vi "Read Data Type Handler Type.vi"(11 "ITest Executive Builder Dialog in":refnum<class "ITest Executive Builder Dialog.lvclass">) -> (3 "ITest Executive Builder Dialog out":refnum<class "ITest Executive Builder Dialog.lvclass">, 4 "Data Type Handler":refnum<class "Test Executive Builder Data Type Handler.lvclass">)   [LabVIEW 2017, in "ITest Executive Builder Dialog.lvclass"]
uses:
  ITest Executive Builder Dialog.lvclass
  Data Type Handler/Test Executive Builder Data Type Handler.lvclass
  ITest Executive Builder Dialog.lvclass/ITest Executive Builder Dialog.ctl
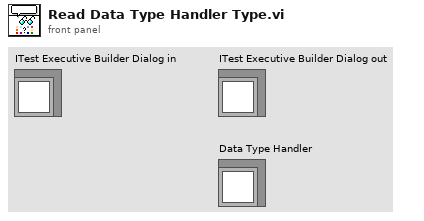
[diagram p1: front panel]
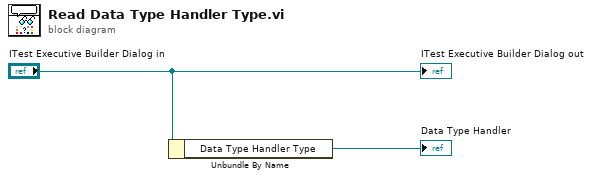
[diagram p0: block diagram]
diagram:
  n1 = Unbundle By Name("ITest Executive Builder Dialog in") -> ("Data Type Handler Type"=→"Data Type Handler":refnum<class "Test Executive Builder Data Type Handler.lvclass">)
  "ITest Executive Builder Dialog out" <- "ITest Executive Builder Dialog in"
